vi "幅频特性.vi"(1 "file path (dialog if empty)":path) -> ()   [LabVIEW 2010]
uses:
  <vilib>/Utility/file.llb/Read From Spreadsheet File (DBL).vi
panel:
  in  "返回":bool
  out "幅频特性曲线":cluster{"all rows":dbl[], "all rows":dbl[]}(graph)
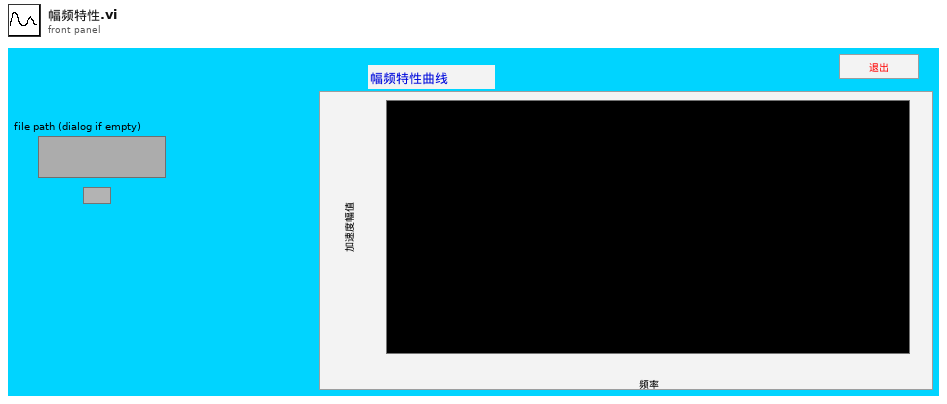
[diagram p1: front panel]
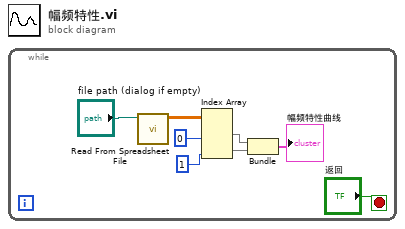
[diagram p0: block diagram]
diagram:
  n1 = while {
    stop <- "返回" stop-if-true
    n2 = call-poly <vilib>:"Read From Spreadsheet File.vi"("file path (dialog if empty)"="file path (dialog if empty)") -> ("all rows"=w8:dbl[][])  [unwired: 6 in, 4 out]
    n3 = Index Array(array=w8, index (col) #1=0 ("disabled index (col)"), index (col) #2=1 ("index (col)")) -> (element #1=w5:dbl[], element #2=w4:dbl[])  [unwired: 2 in]
    n4 = Bundle("all rows"=w5, "all rows"=w4) -> (→"幅频特性曲线":cluster{"all rows":dbl[], "all rows":dbl[]})  [unwired: 1 in]
  }
